vi "F to C.vi"() -> ()   [LabVIEW 2020]
panel:
  out "b/w 35 and 40":i32
  out "Celcius<40":i32
  out "Celcius>40":i32
  in  "stop":bool
  in  "Degree F":dbl
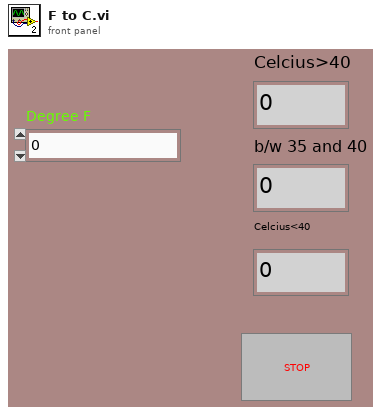
[diagram p1: front panel]
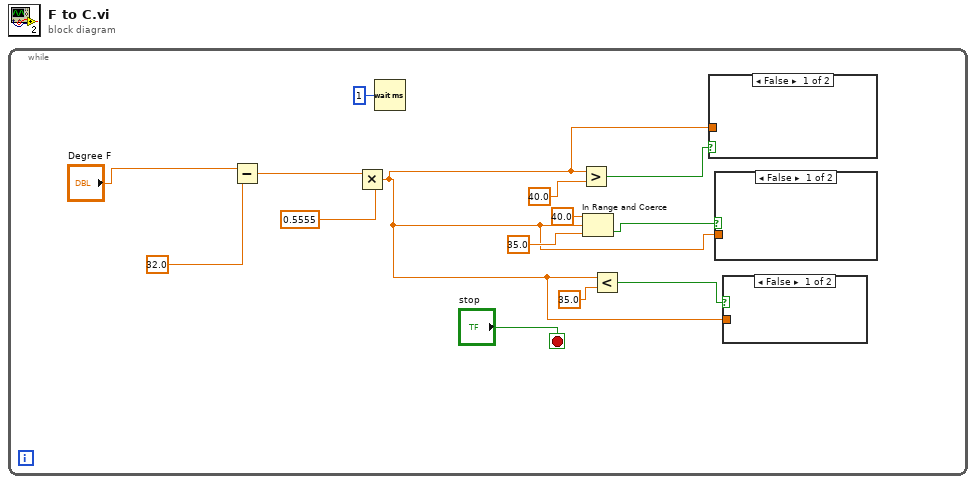
[diagram p0: block diagram]
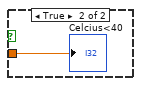
[diagram p2: hidden frame]
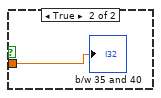
[diagram p3: hidden frame]
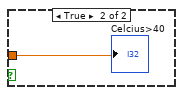
[diagram p4: hidden frame]
diagram:
  n1 = while {
    stop <- "stop" stop-if-true
    n2 = Subtract(x="Degree F", y=32.0 ("Numeric")) -> (x-y=w11:dbl)
    n3 = Multiply(x=w11, y=0.5555 ("Numeric 2")) -> (x*y=w1:dbl)
    n4 = Wait (ms)(milliseconds to wait=u32 1) -> ()  [unwired: 1 out]
    n5 = Greater?(x=w1, y=40.0 ("x")) -> (0:w6:bool)
    n6 = In Range and Coerce(upper limit=40.0, x=w1, lower limit=35.0) -> (In Range?=w4:bool)  [unwired: 1 out]
    n7 = Less?(x=w1, y=35.0 ("x")) -> (x < y?=w5:bool)
    n8 = case shown="False" w6 {
      tunnel: w1 -> [_ w17]
      frame False {
      }
      frame True {
        "Celcius>40" <- w17
      }
    }
    n9 = case shown="False" w4 {
      tunnel: w1 -> [_ w16]
      frame False {
      }
      frame True {
        "b/w 35 and 40" <- w16
      }
    }
    n10 = case shown="False" w5 {
      tunnel: w1 -> [_ w15]
      frame False {
      }
      frame True {
        "Celcius<40" <- w15
      }
    }
  }
